vi "Global Resources.vi"() -> ()   [LabVIEW 2023, in "HAF.lvlib"]
uses:
  All Message Queues.ctl
  Message.ctl
  All Events.ctl
  Stop Event.ctl
  Event Data.ctl
  Pause Event.ctl
  Resume Event.ctl
  Done Event.ctl
  HAF.lvlib
panel:
  in  "Events":T1
  in  "Message Queues":T6
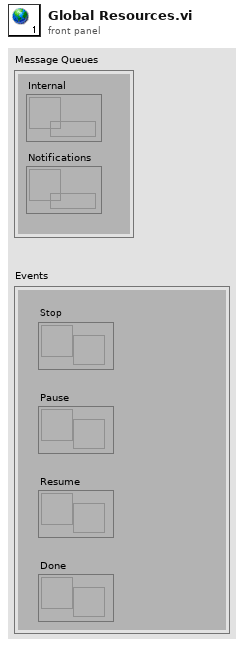
[diagram p1: front panel]
types:
  T1 = typedef "HAF.lvlib/All Events.ctl" = cluster{"Stop":T2, "Pause":T3, "Resume":T4, "Done":T5}
  T2 = typedef "HAF.lvlib/Stop Event.ctl" = refnum<user-event>
  T3 = typedef "HAF.lvlib/Pause Event.ctl" = refnum<user-event>
  T4 = typedef "HAF.lvlib/Resume Event.ctl" = refnum<user-event>
  T5 = typedef "HAF.lvlib/Done Event.ctl" = refnum<user-event>
  T6 = typedef "HAF.lvlib/All Message Queues.ctl" = cluster{"Internal":refnum<queue>, "Notifications":refnum<queue>}
diagram:
